vi "coding(9600).vi"(7 "Кадр на вход\nкодера":bool[](array[boolean])) -> (8 "Поток кодированных \nбитов":bool[](array[boolean]))   [LabVIEW 2013]
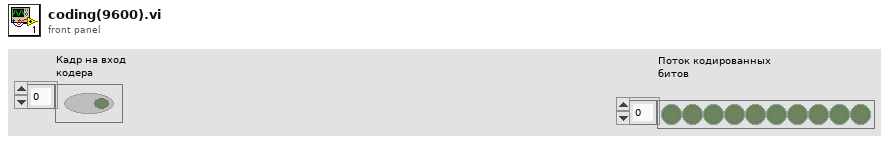
[diagram p1: front panel]
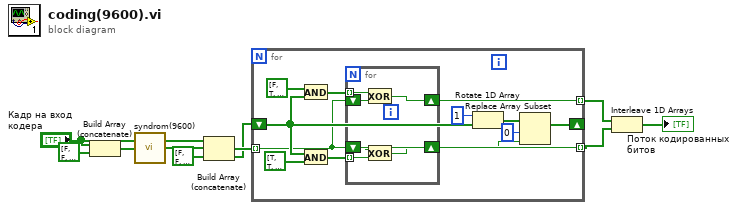
[diagram p0: block diagram]
diagram:
  w3 = bool[] [FALSE, FALSE, FALSE, FALSE, FALSE, FALSE, FALSE, FALSE] ("array")
  n1 = Build Array (concatenate)("Кадр на вход\nкодера", bool[] [FALSE, FALSE, FALSE, FALSE, FALSE, FALSE, FALSE, FALSE, FALSE, FALSE, FALSE, FALSE] ("array")) -> (w6:bool[])
  n2 = call "syndrom(9600).vi"("Кадр для  вычисления \nсиндрома"=w6) -> ("Синдром"=w7:bool[])  [unwired: 14 in]
  n3 = Build Array (concatenate)("Кадр на вход\nкодера", w7, w3) -> (w9:bool[])
  n4 = for {
    tunnel: w9 -> [w10] mode=indexing
    shift-right: [w12] -> _
    shift-left: w3 -> [w11]
    tunnel: [w17] -> w4 mode=indexing
    tunnel: [w16] -> w2 mode=indexing
    n5 = And(x=bool[] [FALSE, TRUE, TRUE, TRUE, FALSE, FALSE, FALSE, TRUE], y=w11) -> (x .and. y?=w19:bool[])
    n6 = And(x=w11, y=bool[] [TRUE, TRUE, TRUE, FALSE, TRUE, FALSE, TRUE, TRUE]) -> (x .and. y?=w18:bool[])
    n7 = for {
      tunnel: w19 -> [w27] mode=indexing
      tunnel: w18 -> [w26] mode=indexing
      shift-right: [w25] -> w17
      shift-left: w10 -> [w24]
      shift-right: [w23] -> w16
      shift-left: w10 -> [w22]
      n8 = Exclusive Or(1:w24, 2:w27) -> (0:w25:bool)
      n9 = Exclusive Or(1:w26, 2:w22) -> (0:w23:bool)
    }
    n10 = Rotate 1D Array(1:w11, 2:1 ("n")) -> (0:w14:bool[])
    n11 = Replace Array Subset(array=w14, new element=w10, index=0) -> (w12:bool[])
  }
  n12 = Interleave 1D Arrays(w4, w2) -> (→"Поток кодированных \nбитов":bool[])
